vi "Example_MoveWithVelocity.vi"() -> ()   [LabVIEW 2018]
doc: "Example how to do a velocity movement. Before starts this example the device must be tuned and the parameter settings must be correct.\nThe example shows:\n - how to initialise and close an interface (e.g. RS232)\n - start of a velocity movement with correct operation mode\n - wait until the target velocity is reached (e.g. 5 seconds)"
panel:
  in  "timeout":u32=1000
  in  "velocity profile":T1={"profileAcceleration"=10000, "profileDeceleration"=10000}
  in  "communication settings in":T2={"deviceName"="EPOS2", "protocolStackName"="MAXON SERIAL V2", "interfaceName"="USB", "portName"="USB0", "baudrate"=1000000, "timeout"=500}
  in  "milliseconds to wait":u32=5000
  in  "targetVelocity":i32=300
  in  "nodeId":u16=1
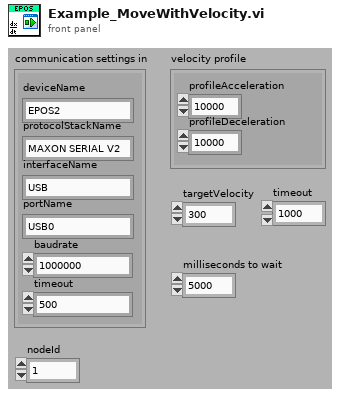
[diagram p1: front panel]
types:
  T1 = cluster{"profileAcceleration":u32, "profileDeceleration":u32}
  T2 = cluster{"deviceName":string, "protocolStackName":string, "interfaceName":string, "portName":string, "baudrate":u32, "timeout":u32}
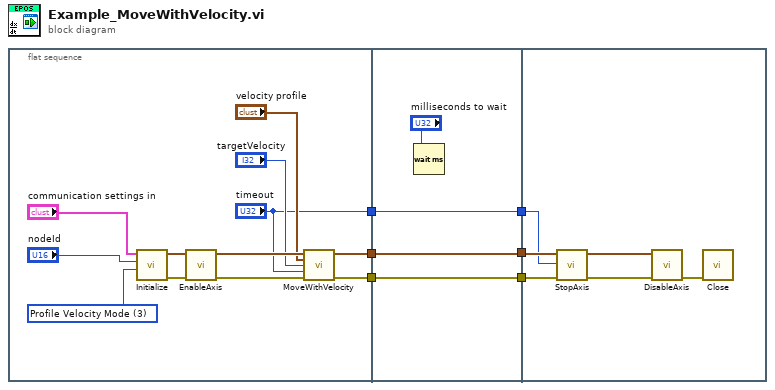
[diagram p0: block diagram]
diagram:
  n1 = flat-sequence {
    tunnel: [w13] -> w5
    tunnel: [w10] -> w3
    tunnel: ["timeout"] -> w2
    tunnel: [w21] -> w6
    tunnel: w5 -> [w21]
    tunnel: [w20] -> w4
    tunnel: w3 -> [w20]
    tunnel: w2 -> [w19]
    tunnel: [w19] -> w1
    tunnel: w6 -> [w27]
    tunnel: w4 -> [w25]
    tunnel: w1 -> [w23]
    frame #0 {
      w16 = i8 3 items=["Profile Position Mode"=1, "Profile Velocity Mode"=3, "Homing Mode"=6, "Interpolated Position Mode"=7, "Position Mode"=-1, "Velocity Mode"=-2, "Current Mode"=-3, "Master Encoder Mode"=-5, "Step Direction Mode"=-6] ("modes of operations")
      n2 = call "Initialize.vi"("modes of operations"=w16, "nodeId"="nodeId", "communication settings in"="communication settings in") -> ("error out"=w15:errorcluster, "axis out"=w12:cluster{"keyHandle":u32, "nodeId":u16})  [unwired: 7 in]
      n3 = call "EnableAxis.vi"("error in (no error)"=w15, "axis in"=w12) -> ("error out"=w14:errorcluster, "axis out"=w11:cluster{"keyHandle":u32, "nodeId":u16})  [unwired: 4 in]
      n4 = call "MoveWithVelocity.vi"("axis in"=w11, "velocity profile"="velocity profile", "targetVelocity"="targetVelocity", "timeout"="timeout", "error in (no error)"=w14) -> ("axis out"=w10:cluster{"keyHandle":u32, "nodeId":u16}, "error out"=w13:errorcluster)  [unwired: 9 in]
    }
    frame #1 {
      n5 = Wait (ms)(milliseconds to wait="milliseconds to wait") -> ()  [unwired: 1 out]
    }
    frame #2 {
      n6 = call "StopAxis.vi"("error in (no error)"=w27, "timeout"=w23, "axis in"=w25) -> ("error out"=w26:errorcluster, "axis out"=w24:cluster{"keyHandle":u32, "nodeId":u16})  [unwired: 3 in]
      n7 = call "DisableAxis.vi"("error in (no error)"=w26, "axis in"=w24) -> ("error out"=w28:errorcluster)  [unwired: 4 in, 1 out]
      n8 = call "Close.vi"("error in (no error)"=w28) -> ()  [unwired: 10 in, 1 out]
    }
  }
